vi "Hysteresis_graph.vi"() -> ()   [LabVIEW 2021]
uses:
  CALIBRATION.lvlib
  <vilib>/ptbypt/NI_PtbyPt.lvlib
panel:
  out "abs_DELTA":dbl[](array[numeric])
  in  "Salita":dbl[][](array[numeric])
  in  "Discesa":dbl[][](array[numeric])
  out "incertezza discesa":dbl
  out "incertezza salita":dbl
  out "incertezza_composta":dbl
  out "u_a12":dbl[](array[numeric])
  out "u_a22":dbl[](array[numeric])
  out "ari_mean discesa":dbl[](array[numeric])
  out "ari_mean salita":dbl[](array[numeric])
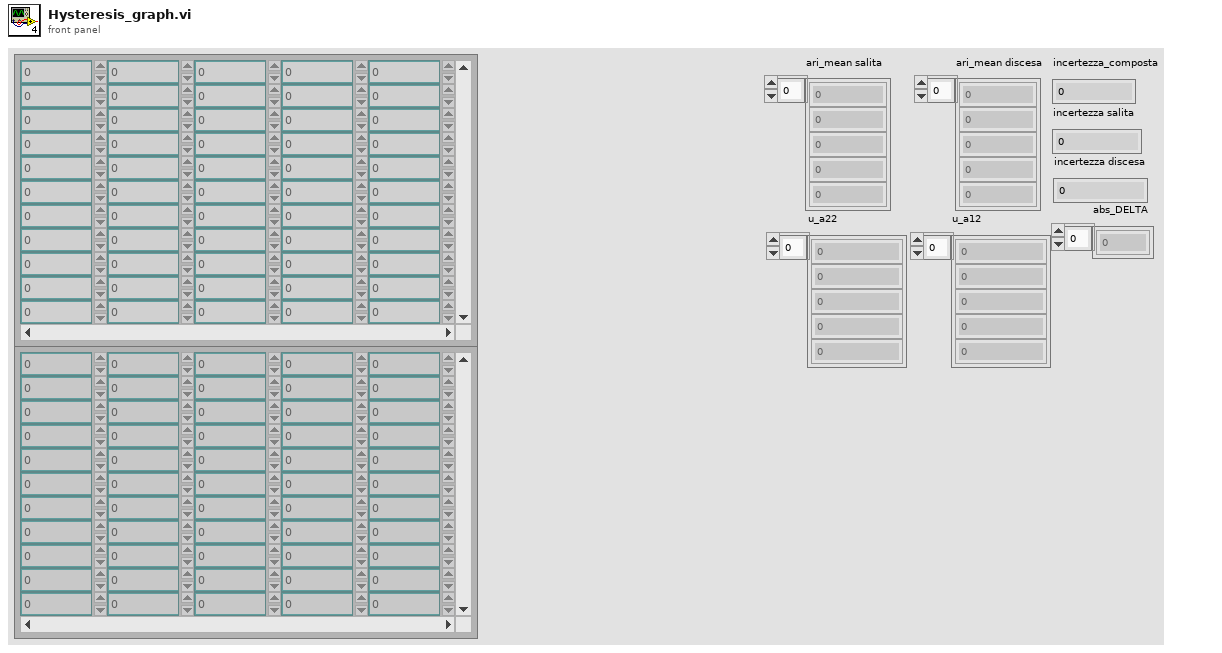
[diagram p1: front panel]
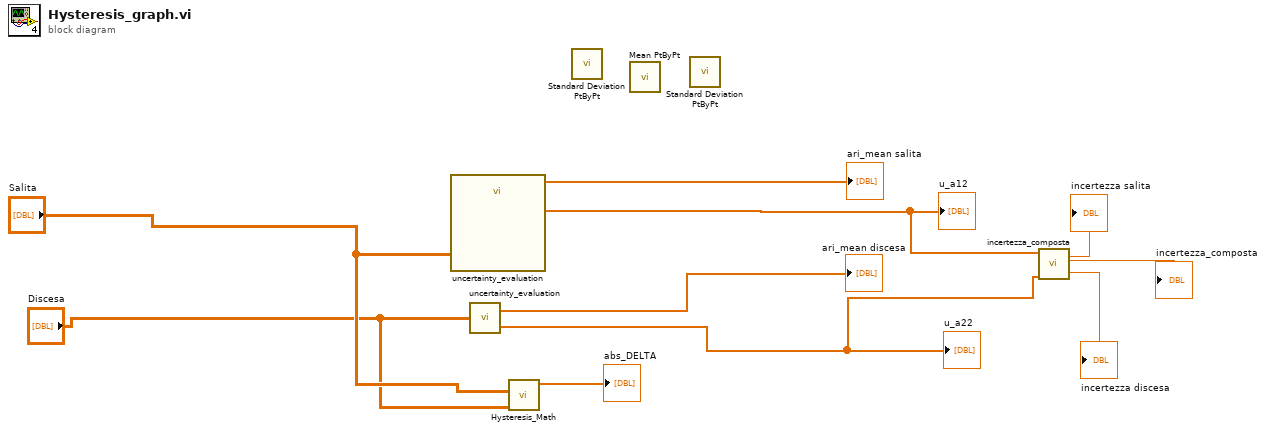
[diagram p0: block diagram]
diagram:
  n1 = call "uncertainty_evaluation.vi"(3:"Salita") -> ("combined_uncertainty"=w8:dbl[], "expected_value"=→"ari_mean salita":dbl[])  [unwired: 2 in]
  "u_a12" <- w8
  n2 = call "uncertainty_evaluation.vi"(3:"Discesa") -> ("combined_uncertainty"=w7:dbl[], "expected_value"=→"ari_mean discesa":dbl[])  [unwired: 2 in]
  "u_a22" <- w7
  n3 = call "Hysteresis_Math.vi"("Discesa"="Discesa", "Salita"="Salita") -> ("abs_DELTA point-by-point"=→"abs_DELTA":dbl[])  [unwired: 2 in, 7 out]
  n4 = call <vilib>:"Standard Deviation PtByPt.vi"() -> ()  [unwired: 3 in, 3 out]
  n5 = call <vilib>:"Mean PtByPt.vi"() -> ()  [unwired: 4 in, 2 out]
  n6 = call <vilib>:"Standard Deviation PtByPt.vi"() -> ()  [unwired: 3 in, 3 out]
  n7 = call "incertezza_composta.vi"("Descending uncertainty point-by-point"=w7, "Ascending uncertainty point-by-point"=w8) -> ("incertezza_composta"=→"incertezza_composta":dbl, "ascending_uncertainty (absolute value)"=→"incertezza discesa":dbl, "descending_uncertainty (absolute value)"=→"incertezza salita":dbl)  [unwired: 7 in]
